vi "Omregn Hex.vi"() -> ()   [LabVIEW 2018]
panel:
  out "Hex [grader]":string
  out "I_Longi direkte grader":dbl
  out "I_Latti direkte grader":dbl
  out "Hex [via rad]":string
  in  "Degrees":dbl
  in  "Lattitude":string="–¼ ×¤<Ã}"
  out "Latti. Grader via rad":dbl
  out "Longi. Grader via rad":dbl
  in  "Longitude":string="–¼ ×¤<Ã}"
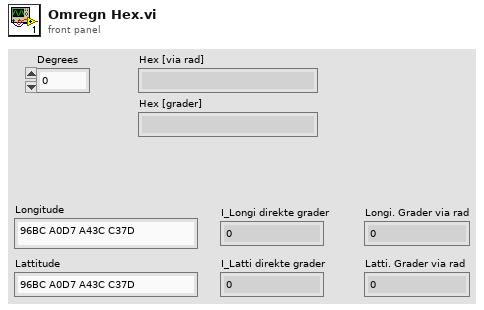
[diagram p1: front panel]
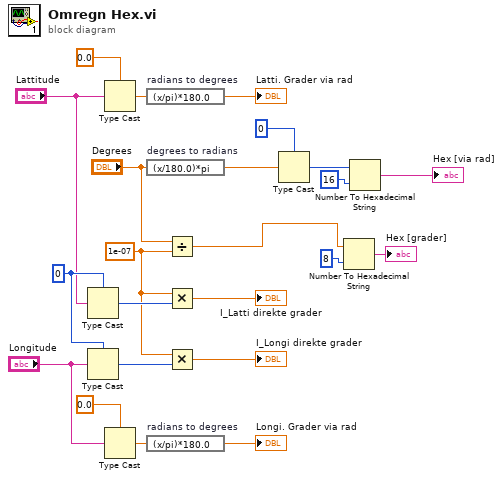
[diagram p0: block diagram]
diagram:
  w5 = 1e-07 ("y")
  w12 = 0
  n1 = Type Cast(type=w12, x="Lattitude") -> (*(type *) &x=w9:i32)
  n2 = Type Cast(type=w12, x="Longitude") -> (*(type *) &x=w7:i32)
  n3 = Type Cast(type=0.0, x="Lattitude") -> (*(type *) &x=w19:dbl)
  n4 = Type Cast(type=0.0, x="Longitude") -> (*(type *) &x=w21:dbl)
  n5 = expression code="(x/pi)*180.0" "radians to degrees"(w19) -> (→"Latti. Grader via rad":dbl)
  n6 = expression code="(x/180.0)*pi" "degrees to radians"("Degrees") -> (w17:dbl)
  n7 = expression code="(x/pi)*180.0" "radians to degrees"(w21) -> (→"Longi. Grader via rad":dbl)
  n8 = Divide(x="Degrees", y=w5) -> (x/y=w1:dbl)
  n9 = Multiply(x=w5, y=w9) -> (x*y=→"I_Latti direkte grader":dbl)
  n10 = Multiply(x=w5, y=w7) -> (x*y=→"I_Longi direkte grader":dbl)
  n11 = Type Cast(type=0, x=w17) -> (*(type *) &x=w15:i32)
  n12 = Number To Hexadecimal String(1:i16 8 ("width (-)"), 2:w1) -> (0:→"Hex [grader]":string)
  n13 = Number To Hexadecimal String(1:i16 16 ("width (-)"), 2:w15) -> (0:→"Hex [via rad]":string)
